vi "Configure Modulation(PSK).vi"(0 "VISA resource name":refnum<visa-resource-name>, 1 "Enable PSK Modulation (F: Disable)":bool, 5 "Channel (1: Channel 1)":i32(ring)=1 items=["Channel 1"=1, "Channel 2"=2], 7 "PSK Source (0: Internal)":i32(ring) items=["Internal", "External"], 9 "Modulating Polarity (0: Positive)":i32(ring) items=["Positive", "Negative"], 11 "error in (no error)":errorcluster, 12 "Phase (180 Degree)":dbl=180.0, 13 "PSK Rate (100 Hz)":dbl=100.0) -> (4 "VISA resource name out":refnum<visa-resource-name>, 15 "error out":errorcluster)   [LabVIEW 2012, in "RIGOL DG4000 Series.lvlib"]
doc: "Configures PSK (Phase Shift Keying) modulation."
uses:
  <instrlib>/RIGOL DG4000 Series/RIGOL DG4000 Series.lvlib
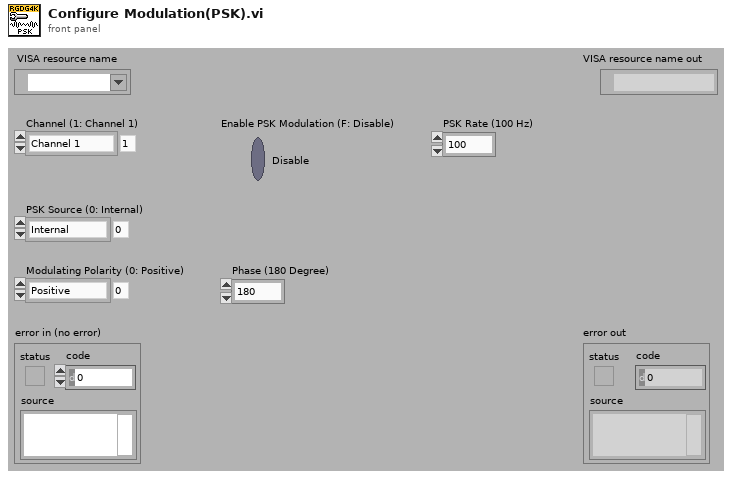
[diagram p1: front panel]
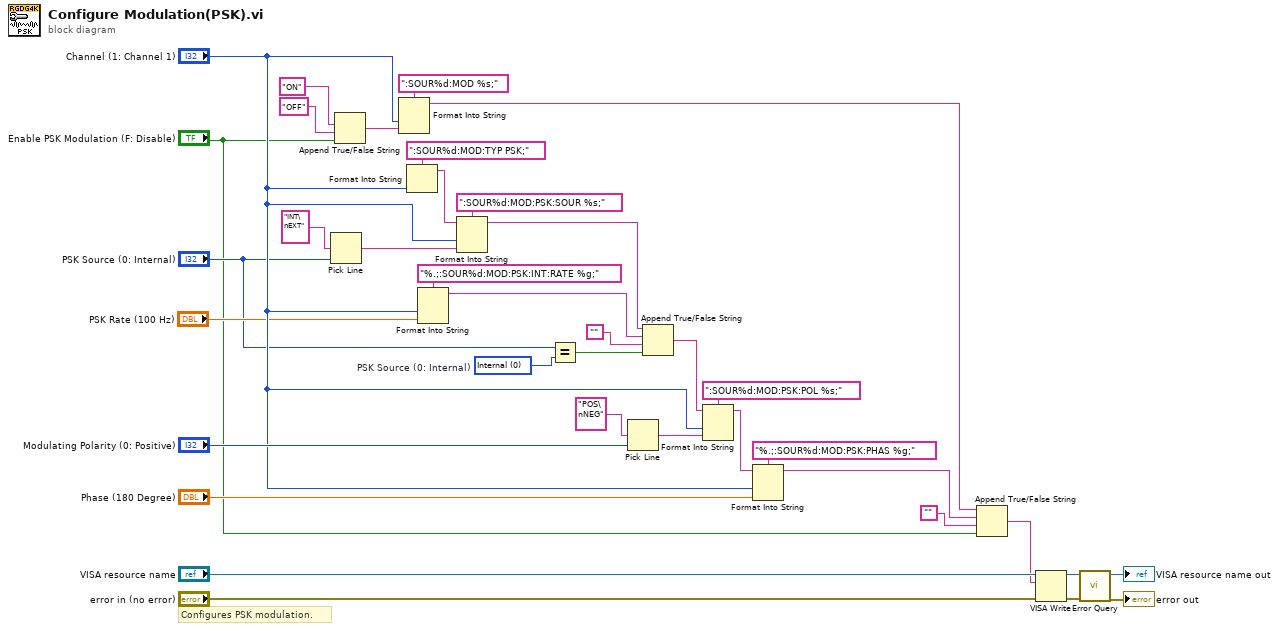
[diagram p0: block diagram]
diagram:
  w8 = 0 items=["Internal", "External"]  # PSK Source (0: Internal)
  # "Configures PSK modulation."
  n1 = Pick Line(multi-line string="INT\nEXT", line index="PSK Source (0: Internal)") -> (output string=w29:string)  [unwired: 1 out]
  n2 = Append True/False String(1:"Enable PSK Modulation (F: Disable)", 2:"OFF", 3:"ON") -> (0:w34:string)  [unwired: 1 out]
  n3 = Format Into String(format string=":SOUR%d:MOD %s;", "Channel (1: Channel 1)", w34) -> (resulting string=w4:string)  [unwired: 2 in, 1 out]
  n4 = Format Into String(format string=":SOUR%d:MOD:TYP PSK;", "Channel (1: Channel 1)") -> (resulting string=w31:string)  [unwired: 2 in, 1 out]
  n5 = Format Into String(format string="%.;:SOUR%d:MOD:PSK:INT:RATE %g;", "Channel (1: Channel 1)", "PSK Rate (100 Hz)") -> (resulting string=w9:string)  [unwired: 2 in, 1 out]
  n6 = Format Into String(format string=":SOUR%d:MOD:PSK:SOUR %s;", initial string=w31, "Channel (1: Channel 1)", w29) -> (resulting string=w10:string)  [unwired: 1 in, 1 out]
  n7 = Equal?(x="PSK Source (0: Internal)", y=w8) -> (x = y?=w11:bool)
  n8 = Pick Line(multi-line string="POS\nNEG", line index="Modulating Polarity (0: Positive)") -> (output string=w25:string)  [unwired: 1 out]
  n9 = Append True/False String(1:w11, 2:"", 3:w9, 4:w10) -> (0:w6:string)
  n10 = Format Into String(format string=":SOUR%d:MOD:PSK:POL %s;", initial string=w6, "Channel (1: Channel 1)", w25) -> (resulting string=w24:string)  [unwired: 1 in, 1 out]
  n11 = Format Into String(format string="%.;:SOUR%d:MOD:PSK:PHAS %g;", initial string=w24, "Channel (1: Channel 1)", "Phase (180 Degree)") -> (resulting string=w3:string)  [unwired: 1 in, 1 out]
  n12 = Append True/False String(1:"Enable PSK Modulation (F: Disable)", 2:"", 3:w3, 4:w4) -> (0:w1:string)
  n13 = VISA Write(VISA resource name="VISA resource name", write buffer=w1, error in (no error)="error in (no error)") -> (VISA resource name out=w18:refnum<visa-resource-name>, error out=w17:errorcluster)  [unwired: 1 out]
  n14 = call <instrlib>:"Error Query.vi"("error in (no error)"=w17, "VISA resource name"=w18) -> ("error out"=→"error out":errorcluster, "VISA resource name out"=→"VISA resource name out":refnum<visa-resource-name>)  [unwired: 8 out]
